vi "sGet NIST Time.vi"(0 "IP Address of NIST Server":string="132.163.4.102", 1 "error in (no error)":errorcluster) -> (2 "NTP Time":u64, 3 "time stamp":timestamp format="^%<%I:%M %p\n%d/%m/%y>T", 4 "error out":errorcluster)   [LabVIEW 2014]
panel:
  out "Used local time generation":bool
  out "raw data":string
  # "This is a first draft to query an NTP server (proof of concept).\nhttp://forums.ni.com/ni/board/message?board.id=170&message.id=458949&jump=true"
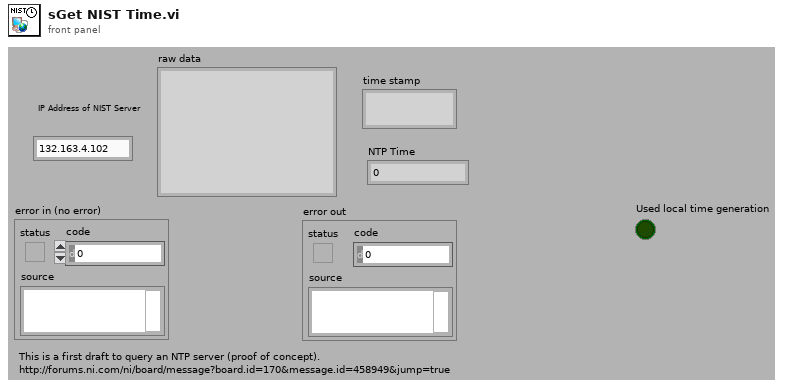
[diagram p1: front panel]
types:
  T1 = cluster{"LI|VM|Mode":u8, "Stratum":u8, "Poll":u8, "Precision":u8, "Root Delay":u32, "Root Dispersion":u32, "Reference Identifier":u32, "Reference Timestamp":fxp<+,64,32>, "Originate Timestamp":fxp<+,64,32>, "Receive Timestamp":fxp<+,64,32>, "Transmit Timestamp":fxp<+,64,32>, "Key Identifier":u32, "Message Digest-1":u64, "Message Digest-2":u64}
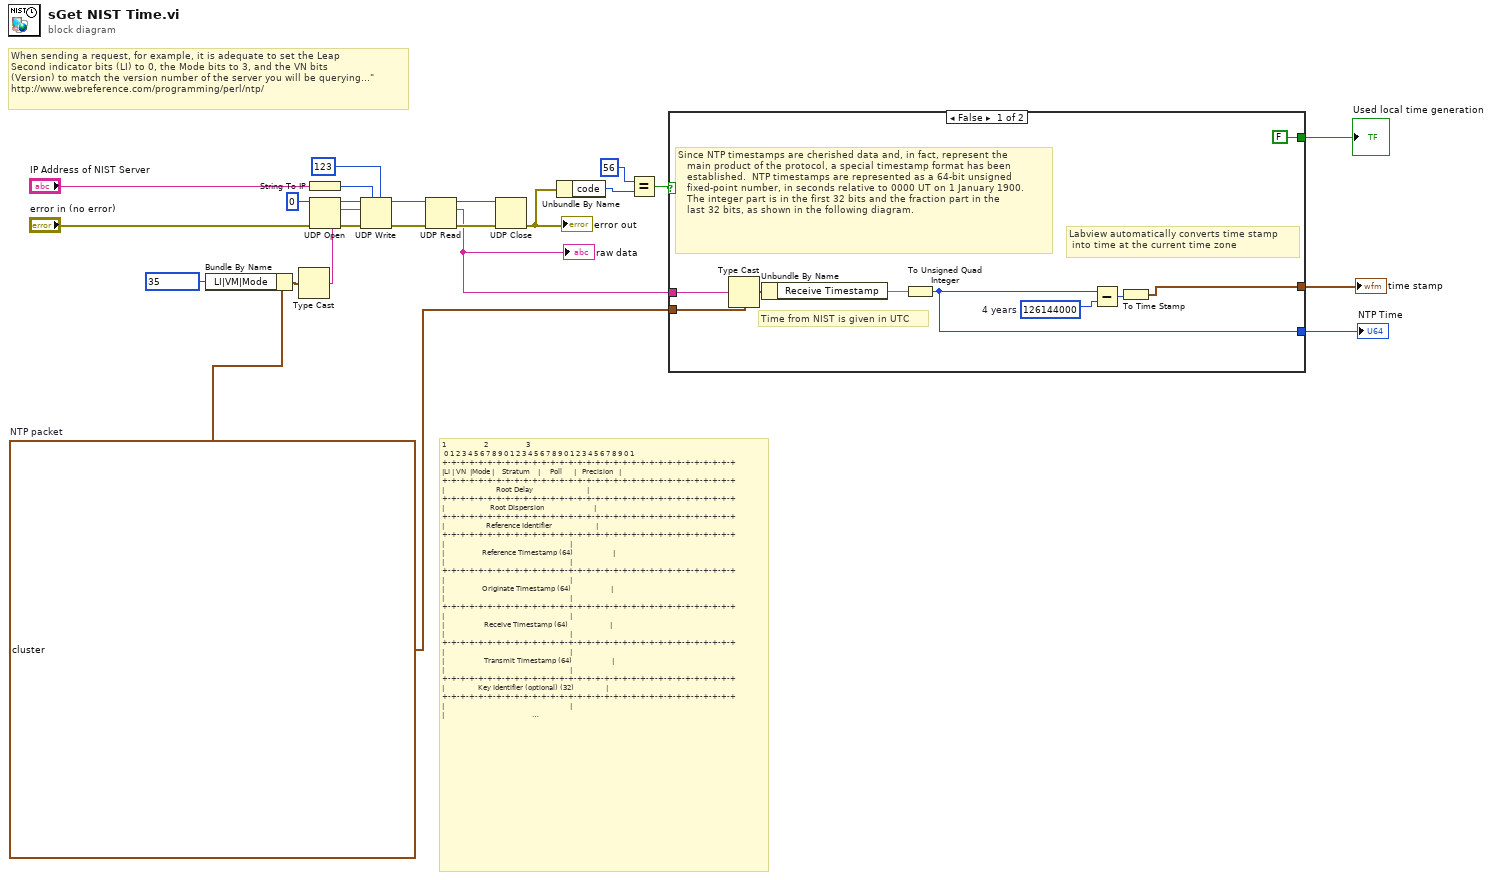
[diagram p0: block diagram]
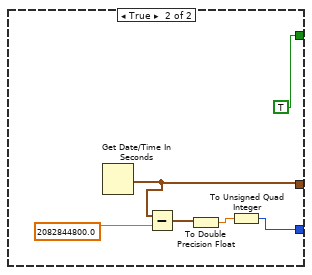
[diagram p2: hidden frame]
diagram:
  w11 = T1 {"LI|VM|Mode"=0, "Stratum"=0, "Poll"=0, "Precision"=0, "Root Delay"=0, "Root Dispersion"=0, "Reference Identifier"=0, "Reference Timestamp"=0.0, "Originate Timestamp"=0.0, "Receive Timestamp"=0.0, "Transmit Timestamp"=0.0, "Key Identifier"=0, "Message Digest-1"=0, "Message Digest-2"=0}  # NTP packet
  # "This is just a simple draft. Verify correct operation!\n\nChristian Altenbach, Nov 2009\naltenbach@gmail.com"
  # "When sending a request, for example, it is adequate to set the Leap\nSecond indicator bits (LI) to 0, the Mode bits to 3, and the VN bits\n(Version) to match the version number of the server you will be querying...\"\nhttp://www.webreference.com/programming/perl/ntp/"
  # "1                   2                   3\n 0 1 2 3 4 5 6 7 8 9 0 1 2 3 4 5 6 7 8 9 0 1 2 3 4 5 6 7 8 9 0 1\n+-+-+-+-+-+-+-+-+-+-+-+-+-+-+-+-+-+-+-+-+-+-+-+-+-+-+-+-+-+-+-+-+\n|LI | VN  |Mode |    Stratum    |     Poll      |   Precision   |\n+-+-+-+-+-+-+-+-+-+-+-+-+-+-+-+-+-+-+-+-+-+-+-+-+-+-+-+-+-+-+-+-+\n|                          Root Delay                           |\n+-+-+-+-+-+-+-+-+-+-+-+-+-+-+-+-+-+-+-+-+-+-+-+-+-+-+-+-+-+-+-+-+\n|                       Root Dispersion                         |\n+-+-+-+-+-+-+-+-+-+-+-+-+-+-+-+-+-+-+-+-+-+-+-+-+-+-+-+-+-+-+-+-+\n|                     Reference Identifier                      |\n+-+-+-+-+-+-+-+-+-+-+-+-+-+-+-+-+-+-+-+-+-+-+-+-+-+-+-+-+-+-+-+-+\n|                                                               |\n|                   Reference Timestamp (64)                    |\n|                                                               |\n+-+-+-+-+-+-+-+-+-+-+-+-+-+-+-+-+-+-+-+-+-+-+-+-+-+-+-+-+-+-+-+-+\n|                                                               |\n|                   Originate Timestamp (64)                    |\n|                                                               |\n+-+-+-+-+-+-+-+-+-+-+-+-+-+-+-+-+-+-+-+-+-+-+-+-+-+-+-+-+-+-+-+-+\n|                                                               |\n|                    Receive Timestamp (64)                     |\n|                                                               |\n+-+-+-+-+-+-+-+-+-+-+-+-+-+-+-+-+-+-+-+-+-+-+-+-+-+-+-+-+-+-+-+-+\n|                                                               |\n|                    Transmit Timestamp (64)                    |\n|                                                               |\n+-+-+-+-+-+-+-+-+-+-+-+-+-+-+-+-+-+-+-+-+-+-+-+-+-+-+-+-+-+-+-+-+\n|                 Key Identifier (optional) (32)                |\n+-+-+-+-+-+-+-+-+-+-+-+-+-+-+-+-+-+-+-+-+-+-+-+-+-+-+-+-+-+-+-+-+\n|                                                               |\n|                                                               |\n|                 Message Digest (optional) (128)               |\n|                                                               |\n|                                                               |\n+-+-+-+-+-+-+-+-+-+-+-+-+-+-+-+-+-+-+-+-+-+-+-+-+-+-+-+-+-+-+-+-+"
  n1 = Bundle By Name(cluster=w11, "LI|VM|Mode"=u8 35) -> (w14:T1)
  n2 = Type Cast(x=w14) -> (*(type *) &x=w17:string)  [unwired: 1 in]
  n3 = String To IP(1:"IP Address of NIST Server") -> (0:w21:u32)
  n4 = UDP Open(8:"error in (no error)", 11:u16 0 ("port")) -> (port=w23:refnum<k16>, 0:w20:errorcluster)  [unwired: 3 in, 1 out]
  n5 = UDP Write(address=w21, port or service name=u16 123, connection ID=w23, data in=w17, 8:w20) -> (error out=w6:errorcluster, 3:w7:refnum<k16>)  [unwired: 1 in]
  n6 = UDP Read(connection ID=w7, 8:w6) -> (data out=w1:string, error out=w4:errorcluster, 3:w5:refnum<k16>)  [unwired: 2 in, 2 out]
  "raw data" <- w1
  n7 = UDP Close(connection ID=w5, 8:w4) -> (error out=w2:errorcluster)  [unwired: 1 out]
  "error out" <- w2
  n8 = Unbundle By Name(w2) -> ("code"=w13:i32)
  n9 = Equal?(x=56, y=w13) -> (x = y?=w3:bool)
  n10 = case shown="False" w3 {
    tunnel: w11 -> [w28 _]
    tunnel: [w27 w38] -> w10
    tunnel: [w26 w34] -> w9
    tunnel: [FALSE ("Used local time generation") TRUE ("Used local time generation")] -> w8
    tunnel: w1 -> [w24 _]
    frame False {
      w31 = u64 126144000  # 4 years
      # "Labview automatically converts time stamp\n into time at the current time zone"
      # "Time from NIST is given in UTC"
      # "Since NTP timestamps are cherished data and, in fact, represent the\n   main product of the protocol, a special timestamp format has been\n   established.  NTP timestamps are represented as a 64-bit unsigned\n   fixed-point number, in seconds relative to 0000 UT on 1 January 1900.\n   The integer part is in the first 32 bits and the fraction part in the\n   last 32 bits, as shown in the following diagram."
      n11 = Type Cast(type=w28, x=w24) -> (*(type *) &x=w29:T1)
      n12 = Unbundle By Name(w29) -> ("Receive Timestamp"=w30:fxp<+,64,32>)
      n13 = To Unsigned Quad Integer(1:w30) -> (0:w26:u64)
      n14 = Subtract(x=w26, y=w31) -> (x-y=w32:u64)
      n15 = To Time Stamp(1:w32) -> (0:w27:timestamp)
    }
    frame True {
      n16 = Get Date/Time In Seconds() -> (seconds since 1Jan1904=w38:timestamp)
      n17 = Subtract(x=w38, y=2082844800.0) -> (x-y=w36:timestamp)
      n18 = To Double Precision Float(number=w36) -> (double precision float=w35:dbl)
      n19 = To Unsigned Quad Integer(1:w35) -> (0:w34:u64)
    }
  }
  "time stamp" <- w10
  "NTP Time" <- w9
  "Used local time generation" <- w8
